vi "Go2XYZ_AlwaysOn (SubVI).vi"(0 ".NET Refnum in":refnum<k24>, 5 "Go to Coordinates":T2={"X [mm]"=25.0, "Y [mm]"=12.5, "Z [mm]"=5.0}, 7 "Axis Speeds":T4={"vX [mm/s]"=25.0, "vY [mm/s]"=12.5, "vZ [mm/s]"=5.0}, 11 "error in (no error)":errorcluster) -> (4 ".NET Refnum out":refnum<k24>, 6 "Final Position":T1, 14 "Initial Position":T3, 15 "error out":errorcluster)   [LabVIEW 2016]
uses:
  C:/Users/Aerotech/Documents/BNLStaveAssembly-blueprint/Bin/Aerotech.A3200.dll
  Bin/Aerotech.A3200.dll
  Motion/MoveAbsMultiple.vi
  Motion/WaitMultiple.vi
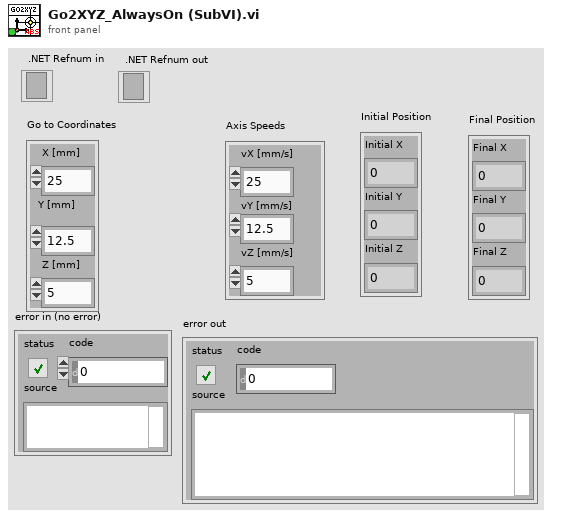
[diagram p1: front panel]
types:
  T1 = cluster{"Final X":dbl, "Final Y":dbl, "Final Z":dbl}
  T2 = cluster{"X [mm]":dbl, "Y [mm]":dbl, "Z [mm]":dbl}
  T3 = cluster{"Initial X":dbl, "Initial Y":dbl, "Initial Z":dbl}
  T4 = cluster{"vX [mm/s]":dbl, "vY [mm/s]":dbl, "vZ [mm/s]":dbl}
  T5 = cluster{"Go to X":dbl, "Go to Y":dbl, "Go to Z":dbl}
  T6 = cluster{"X Position Feedback":dbl, "Y Position Feedback":dbl, "Z Position Feedback":dbl}
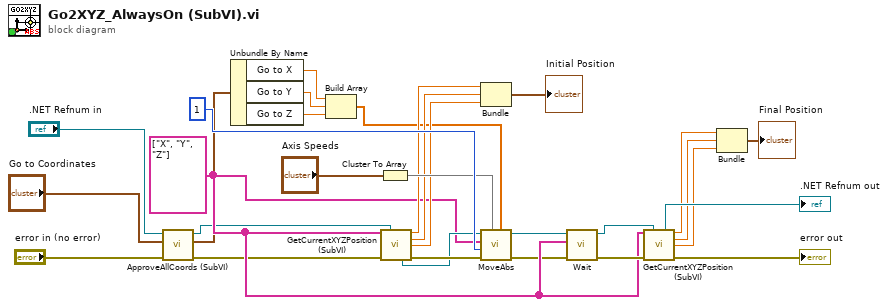
[diagram p0: block diagram]
diagram:
  w18 = string[] ["X", "Y", "Z"]
  n1 = call "ApproveAllCoords (SubVI).vi"("error in (no error)"="error in (no error)", "Go to Coordinates"="Go to Coordinates", "Controller .NET Refnum in"=".NET Refnum in") -> ("error out"=w11:errorcluster, "Approved Coordinates"=w6:T5, "Controller .NET Refnum out"=w7:refnum<k24>)  [unwired: 6 in]
  n2 = Unbundle By Name(w6) -> ("Go to X"=w8:dbl, "Go to Y"=w9:dbl, "Go to Z"=w10:dbl)
  n3 = Build Array(w8, w9, w10) -> (w3:dbl[])
  n4 = Cluster To Array(cluster="Axis Speeds") -> (array=w26:dbl[])
  n5 = call "GetCurrentXYZPosition (SubVI).vi"("Axes Names"=w18, ".NET Refnum in - Device"=w7, "error in (no error)"=w11) -> (".NET Refnum out  - Device"=w28:refnum<k24>, "X Position Feedback"=w25:dbl, "Y Position Feedback"=w24:dbl, "Z Position Feedback"=w23:dbl, "error out"=w29:errorcluster)  [unwired: 7 in, 1 out]
  n6 = Bundle("X Position Feedback"=w25, "Y Position Feedback"=w24, "Z Position Feedback"=w23) -> (→"Initial Position":T6)  [unwired: 1 in]
  n7 = call-poly "MoveAbs.vi"("positions"=w3, "speeds"=w26, "error in (no error)"=w29, "taskId"=1 ("taskNumber"), "axis names"=w18, "controller in"=w28) -> ("error out"=w2:errorcluster, "controller out"=w1:refnum<k24>)  [unwired: 4 in]
  n8 = call-poly "Wait.vi"("error in (no error)"=w2, "axis names"=w18, "controller in"=w1) -> ("error out"=w20:errorcluster, "controller out"=w22:refnum<k24>)  [unwired: 6 in, 1 out]
  n9 = call "GetCurrentXYZPosition (SubVI).vi"("Axes Names"=w18, ".NET Refnum in - Device"=w22, "error in (no error)"=w20) -> (".NET Refnum out  - Device"=→".NET Refnum out":refnum<k24>, "X Position Feedback"=w17:dbl, "Y Position Feedback"=w16:dbl, "Z Position Feedback"=w15:dbl, "error out"=→"error out":errorcluster)  [unwired: 7 in, 1 out]
  n10 = Bundle("X Position Feedback"=w17, "Y Position Feedback"=w16, "Z Position Feedback"=w15) -> (→"Final Position":T6)  [unwired: 1 in]
